vi "RBF Weights.vi"(11 "Array of Double in":dbl[](array[numeric])) -> (2 "Array of Double out":dbl[](array[numeric]), 3 "Array of Double 3":dbl[](array[numeric]))   [LabVIEW 2021]
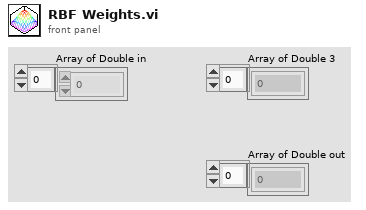
[diagram p1: front panel]
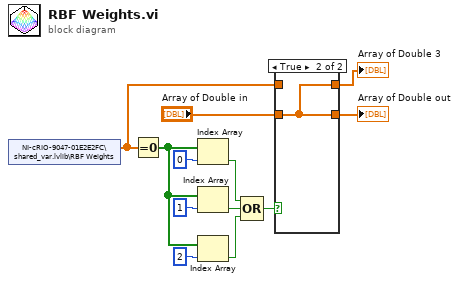
[diagram p0: block diagram]
diagram:
  n1 = shared-variable "NI-cRIO-9047-01E2E2FC\\shared_var.lvlib\\RBF Weights"() -> (w5:dbl[])  [unwired: 1 in, 1 out]
  n2 = Equal To 0?(x=w5) -> (x = 0?=w11:bool[])
  n3 = Index Array(array=w11, index=0) -> (element=w6:bool)
  n4 = Index Array(array=w11, index=1) -> (element=w10:bool)
  n5 = Index Array(array=w11, index=2) -> (element=w12:bool)
  n6 = Compound Arithmetic op=OR(w6, w10, w12) -> (w7:bool)
  n7 = case shown="True" w7 {
    tunnel: [w13 w14] -> w2
    tunnel: "Array of Double in" -> [_ w14]
    tunnel: [w13 w14] -> w4
    tunnel: w5 -> [w13 _]
    frame False {
    }
    frame True {
    }
  }
  "Array of Double out" <- w4
  "Array of Double 3" <- w2
